vi "VI-Get Reg Event Components.vi"(0 "VI in":refnum<vi>, 11 "error in (no error)":errorcluster) -> (4 "VI out":refnum<vi>, 6 "Block Diagram":refnum<vi>, 8 "Components":T1, 15 "error out":errorcluster)   [LabVIEW 2015]
uses:
  VI-Reg Event Components.ctl
  <vilib>/Utility/traverseref.llb/TRef TravTarget.ctl
  <vilib>/Utility/traverseref.llb/VI Scripting - Traverse.lvlib
panel:
  out "Control":refnum<vi>
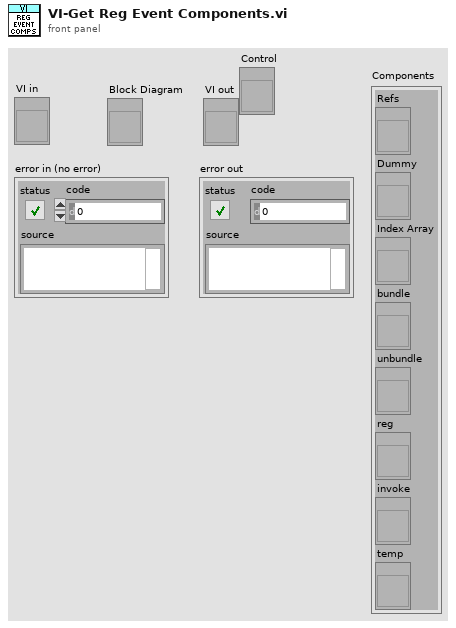
[diagram p1: front panel]
types:
  T1 = typedef "VI-Reg Event Components.ctl" = cluster{"Refs":refnum<vi>, "Dummy":refnum<vi>, "Index Array":refnum<vi>, "bundle":refnum<vi>, "unbundle":refnum<vi>, "reg":refnum<vi>, "invoke":refnum<vi>, "temp":refnum<vi>}
  T2 = typedef "TRef TravTarget.ctl" = enum16{"FP", "BD", "Other"}
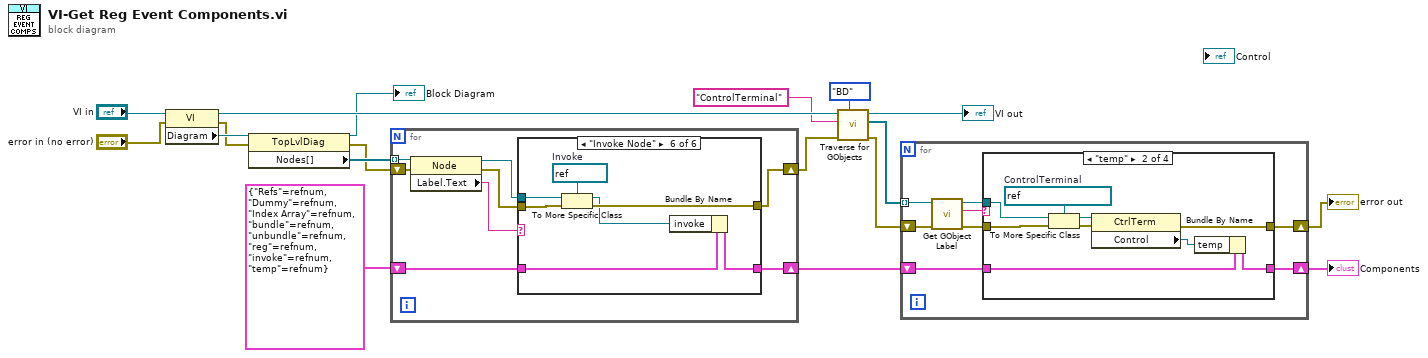
[diagram p0: block diagram]
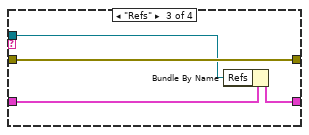
[diagram p3: hidden frame]
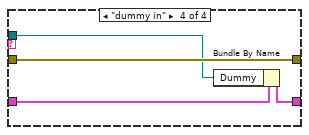
[diagram p4: hidden frame]
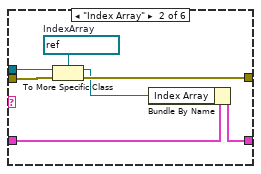
[diagram p6: hidden frame]
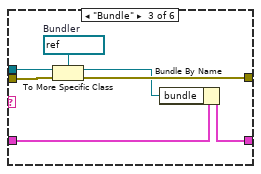
[diagram p7: hidden frame]
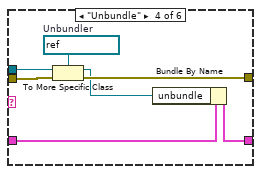
[diagram p8: hidden frame]
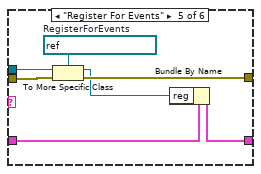
[diagram p9: hidden frame]
diagram:
  n1 = property class="VI"(reference="VI in", error in="error in (no error)") -> (reference out=w11:refnum<vi>, error out=w16:errorcluster, "Diagram"=w17:refnum<vi>)
  n2 = property class="TopLvlDiag"(reference=w17, error in=w16) -> (reference out=→"Block Diagram":refnum<vi>, error out=w13:errorcluster, "Nodes[]"=w14:refnum<vi>[])
  n3 = for {
    tunnel: w14 -> [w26] mode=indexing
    shift-right: [w19] -> w10
    shift-left: w13 -> [w25]
    shift-right: [w22] -> w6
    shift-left: T1 {"Refs"=refnum, "Dummy"=refnum, "Index Array"=refnum, "bundle"=refnum, "unbundle"=refnum, "reg"=refnum, "invoke"=refnum, "temp"=refnum} ("Components") -> [w21]
    n4 = property class="Node"(reference=w26, error in=w25) -> (reference out=w23:refnum<vi>, error out=w20:errorcluster, "Label.Text"=w24:string)
    n5 = case shown="\"Invoke Node\"" w24 {
      tunnel: w23 -> [_ w33 w40 w47 w54 w61]
      tunnel: w21 -> [w28 w35 w42 w49 w56 w63]
      tunnel: [w28 w34 w41 w48 w55 w62] -> w22
      tunnel: w20 -> [w27 w32 w39 w46 w53 w60]
      tunnel: [w27 w31 w38 w45 w52 w59] -> w19
      frame "False", Default {
      }
      frame "Index Array" {
        w30 = refnum<vi> refnum  # IndexArray
        n6 = To More Specific Class(target class=w30, reference=w33, error in=w32) -> (specific class reference=w29:refnum<vi>, error out=w31:errorcluster)
        n7 = Bundle By Name(cluster=w35, "Index Array"=w29) -> (w34:T1)
      }
      frame "Bundle" {
        w37 = refnum<vi> refnum  # Bundler
        n8 = To More Specific Class(target class=w37, reference=w40, error in=w39) -> (specific class reference=w36:refnum<vi>, error out=w38:errorcluster)
        n9 = Bundle By Name(cluster=w42, "bundle"=w36) -> (w41:T1)
      }
      frame "Unbundle" {
        w44 = refnum<vi> refnum  # Unbundler
        n10 = To More Specific Class(target class=w44, reference=w47, error in=w46) -> (specific class reference=w43:refnum<vi>, error out=w45:errorcluster)
        n11 = Bundle By Name(cluster=w49, "unbundle"=w43) -> (w48:T1)
      }
      frame "Register For Events" {
        w51 = refnum<vi> refnum  # RegisterForEvents
        n12 = To More Specific Class(target class=w51, reference=w54, error in=w53) -> (specific class reference=w50:refnum<vi>, error out=w52:errorcluster)
        n13 = Bundle By Name(cluster=w56, "reg"=w50) -> (w55:T1)
      }
      frame "Invoke Node" {
        w58 = refnum<vi> refnum  # Invoke
        n14 = To More Specific Class(target class=w58, reference=w61, error in=w60) -> (specific class reference=w57:refnum<vi>, error out=w59:errorcluster)
        n15 = Bundle By Name(cluster=w63, "invoke"=w57) -> (w62:T1)
      }
    }
  }
  n16 = call <vilib>:"Traverse for GObjects.vi"("Traverse Target"=TRef_TravTarget."BD", "error in (no error)"=w10, "Class Name"="ControlTerminal", "VI Refnum"=w11) -> ("error out"=w3:errorcluster, "References"=w4:refnum<vi>[], "dup VI Refnum"=→"VI out":refnum<vi>)  [unwired: 4 in, 1 out]
  n17 = for {
    shift-right: [w67] -> w5
    shift-left: w6 -> [w68]
    tunnel: w4 -> [w71] mode=indexing
    shift-right: [w64] -> w2
    shift-left: w3 -> [w70]
    n18 = call <vilib>:"Get GObject Label.vi"("error in (no error)"=w70, "GObject"=w71) -> ("error out"=w65:errorcluster, "Object Label"=w69:string, "dup GObject"=w66:refnum<vi>)  [unwired: 5 in, 2 out]
    n19 = case shown="\"temp\"" w69 {
      tunnel: w68 -> [w73 w82 w86 w90]
      tunnel: [w73 w81 w85 w89] -> w67
      tunnel: w66 -> [_ w74 w83 w87]
      tunnel: w65 -> [w72 w77 w84 w88]
      tunnel: [w72 w76 w84 w88] -> w64
      frame "False", Default {
      }
      frame "temp" {
        w79 = refnum<vi> refnum  # ControlTerminal
        n20 = To More Specific Class(target class=w79, reference=w74, error in=w77) -> (specific class reference=w78:refnum<vi>, error out=w80:errorcluster)
        n21 = property class="CtrlTerm"(reference=w78, error in=w80) -> (error out=w76:errorcluster, "Control"=w75:refnum<vi>)  [unwired: 1 out]
        n22 = Bundle By Name(cluster=w82, "temp"=w75) -> (w81:T1)
      }
      frame "Refs" {
        n23 = Bundle By Name(cluster=w86, "Refs"=w83) -> (w85:T1)
      }
      frame "dummy in" {
        n24 = Bundle By Name(cluster=w90, "Dummy"=w87) -> (w89:T1)
      }
    }
  }
  "error out" <- w2
  "Components" <- w5
